vi "Check For Poly VI.vi"(8 "Error In":errorcluster, 11 "VI Reference":refnum<vi>) -> (0 "Error Out":errorcluster, 1 "Dependency Paths":path[](array[path]), 2 "Poly VI?":bool, 3 "VI Reference":refnum<vi>)   [LabVIEW 2014]
panel:
  out "Dependency Names":string[](array[string])
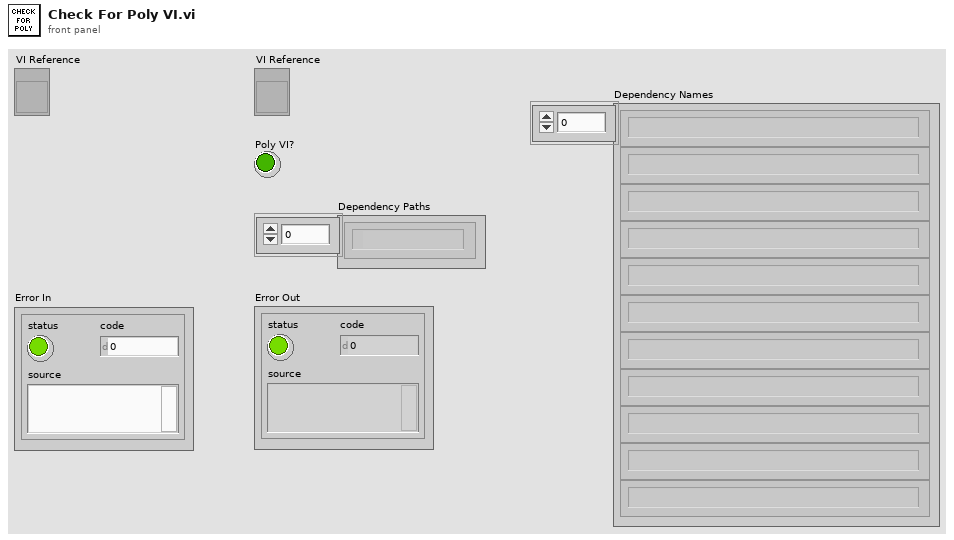
[diagram p1: front panel]
types:
  T1 = enum32{"invalid VI type", "Standard VI", "Control VI", "Global VI", "Polymorphic VI", "Configuration VI", "SubSystem", "Facade VI", "Method VI", "Statechart Diagram VI"}
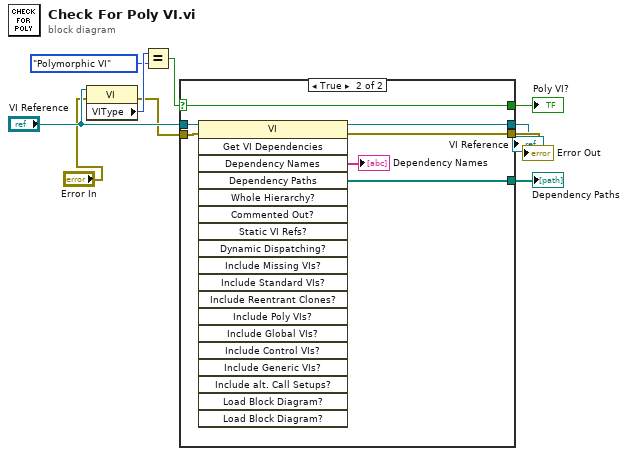
[diagram p0: block diagram]
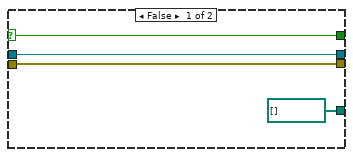
[diagram p2: hidden frame]
diagram:
  n1 = property class="VI"(reference="VI Reference", error in="Error In") -> (error out=w4:errorcluster, "VIType"=w10:T1)  [unwired: 1 out]
  n2 = Equal?(x=w10, y=T1."Polymorphic VI" ("VI Type")) -> (x = y?=w8:bool)
  n3 = case shown="True" w8 {
    selector: w8 -> [w13 w19]
    tunnel: "VI Reference" -> [w12 w21]
    tunnel: [w13 w19] -> w7
    tunnel: [path[] [] ("Dependency Paths") w18] -> w5
    tunnel: w4 -> [w11 w17]
    tunnel: [w11 w16] -> w3
    tunnel: [w12 w15] -> w1
    frame False {
    }
    frame True {
      n4 = invoke class="VI" method="Get VI Dependencies"(reference=w21, error in=w17) -> (reference out=w15:refnum<vi>, error out=w16:errorcluster, "Dependency Names"=→"Dependency Names":string[], "Dependency Paths"=w18:path[])  [unwired: 17 in, 15 out]
    }
  }
  "Poly VI?" <- w7
  "Dependency Paths" <- w5
  "Error Out" <- w3
  "VI Reference" <- w1
